vi "Close.vi"   [LabVIEW 2017, in "NI_XML.lvlib"]
doc: "Closes a reference for all XML parser classes. You can use this polymorphic VI to close refnums from the NamedNodeMap class, the NodeList class, the Implementation class, or the Node class. The Node class encompasses all other XML classes."
uses:
  <vilib>/xml/NI_XML.lvlib
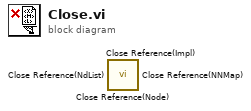
[diagram p0: block diagram]
diagram:
  n1 = call <vilib>:"Close Reference(Node).vi"() -> ()  [unwired: 9 in, 1 out]
  n2 = call <vilib>:"Close Reference(Impl).vi"() -> ()  [unwired: 9 in, 1 out]
  n3 = call <vilib>:"Close Reference(NdList).vi"() -> ()  [unwired: 9 in, 1 out]
  n4 = call <vilib>:"Close Reference(NNMap).vi"() -> ()  [unwired: 9 in, 1 out]
